vi "SwitchBoard_IVCV.vi"(8 "error in":errorcluster, 10 "Measurement type":enum16{"IV", "CV", "Debug", "Test_contact"}(ring)=enum."Debug", 11 "Handle":u32) -> (0 "error out":errorcluster, 3 "Handle out":u32)   [LabVIEW 2016]
doc: "Set IV or CV configuration on switchboard."
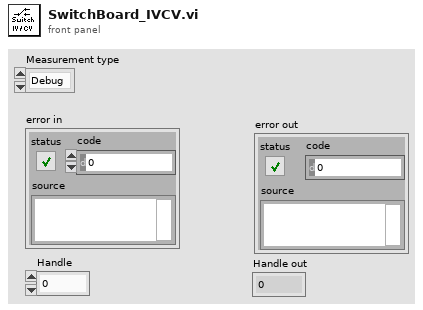
[diagram p1: front panel]
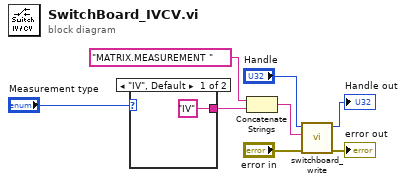
[diagram p0: block diagram]
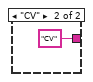
[diagram p2: hidden frame]
diagram:
  n1 = case shown="\"IV\", Default" "Measurement type" {
    tunnel: ["IV" ("string") "CV" ("string")] -> w2
    frame "IV", Default {
    }
    frame "CV" {
    }
  }
  n2 = Concatenate Strings("MATRIX.MEASUREMENT " ("string"), w2) -> (w7:string)
  n3 = call <instrlib>:"switchboard_write.vi"("error in"="error in", "Buffer"=w7, "Handle"="Handle") -> ("error out"=→"error out":errorcluster, "Handle"=→"Handle out":u32)  [unwired: 6 in, 1 out]
